vi "test_pushdata_singleperiod.vi"() -> ()   [LabVIEW 2015]
uses:
  <vilib>/Utility/file.llb/Read From Spreadsheet File (DBL).vi
  <vilib>/functionblocks/Accumulate/Accumulate/Accumulate.vi
  <vilib>/functionblocks/FB Core/FB Core.xnode
  <vilib>/functionblocks/NI_FunctionBlock Libraries.lvlib
  <vilib>/rvi/interface/nirviMethod/nirviMethod.xnode
  <vilib>/FPGAPlugInAG/Dynamic/niLvFpga_WriteFifo_Dynamic.vi
  <vilib>/rvi/errors/niLvFpgaMergeErrorWithErrorCode.vi
panel:
  out "y_final_size":i32
  out "x_final_size":i32
  out "built-up_ref (ramp)":dbl[](graph)
  out "built-up  x_ref(triangle wave)":dbl[](graph)
  out "Empty Elements Remaining":u32
  out "(int) y*floor(x/y)":u64
  out "base y_ref (ramp)":dbl[](graph)
  in  "reference traj path 2":path=path "C:/Users/arnold/Documents/labview/afm_imaging/data/data-in-singleperiod.csv"
  out "points_per_line":i32=250000
  in  "number-of-lines":i32
  out "base x_ref(triangle wave)":dbl[](graph)
  out "elements left 2":i32=1
  out "accumulation 2":dbl format="%#_6f"
  out "x = 0? 2":bool
  out "nsamps 2":i32
  in  "STOP":bool
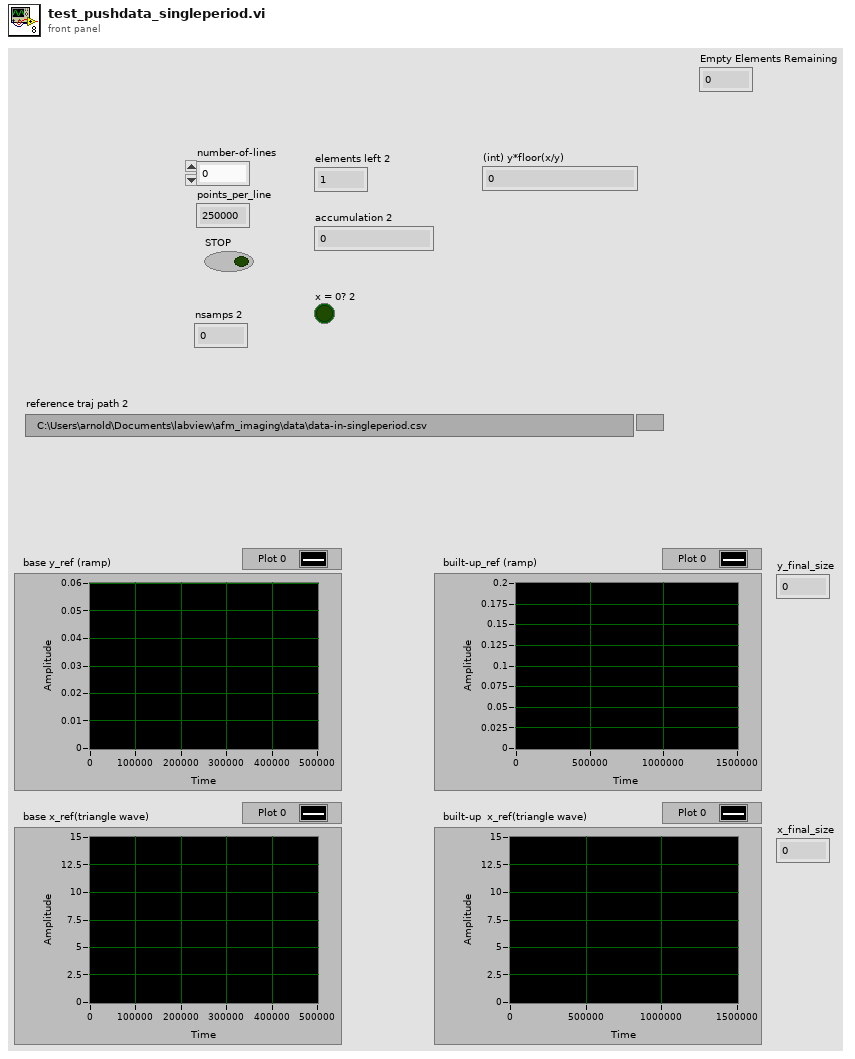
[diagram p1: front panel]
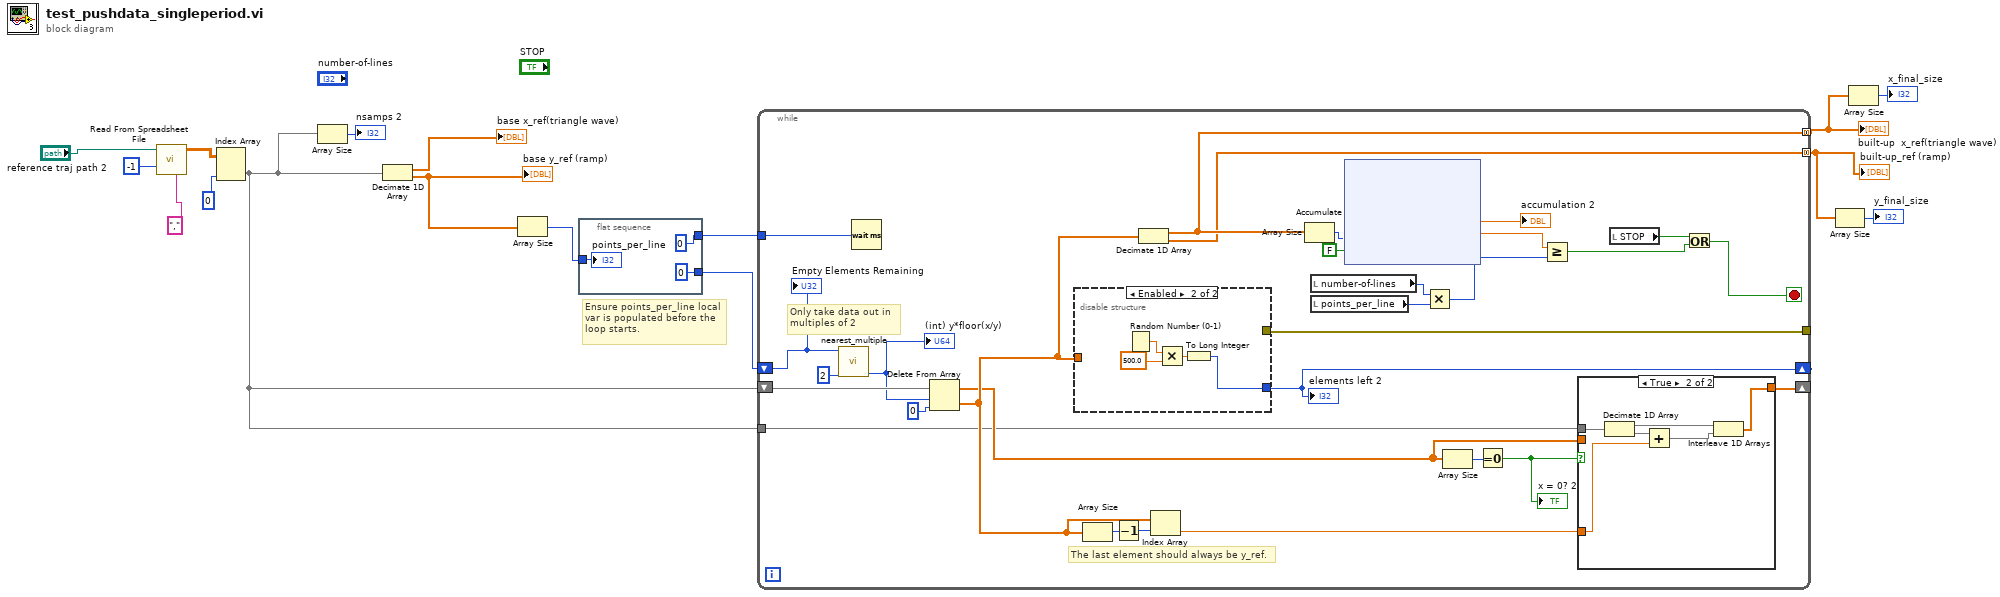
[diagram p0: block diagram]
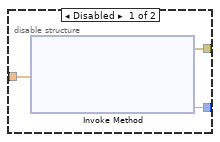
[diagram p3: hidden frame]
diagram:
  # "Ensure points_per_line local\nvar is populated before the\nloop starts."
  n1 = call-poly <vilib>:"Read From Spreadsheet File.vi"("delimiter (\\t)"=",", "number of rows (all:-1)"=-1, "file path (dialog if empty)"="reference traj path 2") -> ("all rows"=w8:dbl[][])  [unwired: 4 in, 4 out]
  n2 = Index Array(array=w8, index (col)=0 ("dimension size")) -> (element=w7:dbl[])  [unwired: 1 in]
  n3 = Array Size(array=w7) -> (size(s)=→"nsamps 2":i32)
  n4 = Decimate 1D Array(w7) -> (→"base x_ref(triangle wave)":dbl[], w5:dbl[])
  "base y_ref (ramp)" <- w5
  n5 = Array Size(array=w5) -> (size(s)=w15:i32)
  n6 = flat-sequence {
    tunnel: w15 -> [w17]
    tunnel: [0] -> w14
    tunnel: [u32 0 ("Empty Elements Remaining")] -> w13
    frame #0 {
      "points_per_line" <- w17
    }
  }
  n7 = while {
    tunnel: w14 -> [w47]
    shift-right: [w45] -> _
    shift-left: w13 -> [w36]
    shift-right: [w26] -> _
    shift-left: w7 -> [w46]
    tunnel: w7 -> [w23]
    tunnel: [w30] -> _
    tunnel: [w21] -> w4 mode=concatenating
    tunnel: [w20] -> w1 mode=concatenating
    stop <- w37 stop-if-true
    # "The last element should always be y_ref."
    # "Only take data out in \nmultiples of 2"
    n8 = call "nearest_multiple.vi"("y"=u32 2 ("Empty Elements Remaining"), "x"=w36) -> ("(int) y*floor(x/y)"=w35:u64)  [unwired: 8 in, 1 out]
    "(int) y*floor(x/y)" <- w35
    n9 = Wait (ms)(milliseconds to wait=w47) -> ()  [unwired: 1 out]
    n10 = Delete From Array(array=w46, length=w35, index=0) -> (deleted portion=w27:dbl[], array with subset deleted=w25:dbl[])
    n11 = disable-structure shown="Enabled" {
      disable-tunnel: [w57 w58] -> w45
      disable-tunnel: w27 -> [w56 _]
      disable-tunnel: [w55 _] -> w30
      frame Disabled {
        n12 = xnode "Invoke Method"("Data"=w56) -> ("error out"=w55:errorcluster, "Empty Elements Remaining"=w57:u32)  [unwired: 3 in, 1 out]
      }
      frame Enabled {
        n13 = Random Number (0-1)() -> (number: 0 to 1=w61:dbl)
        n14 = Multiply(x=w61, y=500.0) -> (x*y=w59:dbl)
        n15 = To Long Integer(number=w59) -> (32bit integer=w58:i32)
      }
    }
    "elements left 2" <- w45
    n16 = Array Size(array=w27) -> (size(s)=w28:i32)
    n17 = Decrement(x=w28) -> (x-1=w29:i32)
    n18 = Decimate 1D Array(w27) -> (w21:dbl[], w20:dbl[])
    n19 = Index Array(array=w27, index=w29) -> (element=w22:dbl)
    n20 = Array Size(array=w21) -> (size(s)=w41:i32)
    n21 = local read "number-of-lines"() -> (w33:i32)
    n22 = local read "points_per_line"() -> (w32:i32)
    n23 = xnode "Accumulate"("reset"=FALSE, "input"=w41) -> ("accumulation"=w40:dbl)  [unwired: 2 in, 1 out]
    "accumulation 2" <- w40
    n24 = Multiply(x=w33, y=w32) -> (x*y=w31:i32)
    n25 = Array Size(array=w25) -> (size(s)=w39:i32)
    n26 = Equal To 0?(x=w39) -> (x = 0?=w24:bool)
    "x = 0? 2" <- w24
    n27 = Greater Or Equal?(x=w40, y=w31) -> (x >= y?=w44:bool)
    n28 = case shown="True" w24 {
      tunnel: [w48 w49] -> w26
      tunnel: w25 -> [w48 _]
      tunnel: w23 -> [_ w54]
      tunnel: w22 -> [_ w52]
      frame False {
      }
      frame True {
        n29 = Decimate 1D Array(w54) -> (w51:dbl[], w53:dbl[])
        n30 = Add(x=w53, y=w52) -> (x+y=w50:dbl[])
        n31 = Interleave 1D Arrays(w51, w50) -> (w49:dbl[])
      }
    }
    n32 = local read "STOP"() -> (w38:bool)
    n33 = Or(x=w38, y=w44) -> (x .or. y?=w37:bool)
    "Empty Elements Remaining" <- w36
  }
  "built-up  x_ref(triangle wave)" <- w4
  "built-up_ref (ramp)" <- w1
  n34 = Array Size(array=w1) -> (size(s)=→"y_final_size":i32)
  n35 = Array Size(array=w4) -> (size(s)=→"x_final_size":i32)
